vi "rvc Quadcopter Model.vi"(4 "tpp":dbl[](array[numeric]), 5 "d":dbl, 7 "b":dbl, 8 "omega4":dbl, 9 "omega3":dbl, 10 "omega2":dbl, 11 "omega1":dbl) -> (2 "tpp_2dot 2":dbl[](array[numeric]), 3 "xyz_2dot":dbl[](array[numeric]))   [LabVIEW 2013]
uses:
  <vilib>/imath/engines/lvmath2/RunTimeEngine/ErrorHandling/NIMS_Finalize Error.vi
  <vilib>/imath/engines/lvmath2/RunTimeEngine/Managers/WorkSpace/UID Generator.vi
  <vilib>/imath/engines/lvmath2/RunTimeEngine/Managers/SymbolTable/Clear UID.vi
  <vilib>/imath/engines/lvmath2/RunTimeEngine/NodeEndStatement/NIMS_NodeEndStatement_Output.vi
  <instcachedir>/0/NIMS_NodeEndStatement_Output_53EC0D466D134D7ABD903AC30B43404B.lvgen/NIMS_NodeEndStatement_Output_53EC0D466D134D7ABD903AC30B43404B_001.vi
  <vilib>/imath/engines/lvmath2/RunTimeEngine/RunTimeType/NIMS_RunTimeType_From StrictType (excl LVString).vi
  <instcachedir>/0/NIMS_RunTimeType_From StrictType (excl LVString)_4DEE718D6EB74582AA20236969C084FC.lvgen/NIMS_RunTimeType_From StrictType (excl LVString)_4DEE718D6EB74582AA20236969C084FC_000.vi
  <vilib>/imath/engines/lvmath2/RunTimeEngine/LocalVariableDefStatement/MC_LocalVariableDefStatement_Display.vi
  <vilib>/imath/engines/lvmath2/RunTimeEngine/Managers/SymbolTable/NIMS_WorkSpace.lvlib
panel:
  out "theta":dbl
  out "phi":dbl
  out "psi":dbl
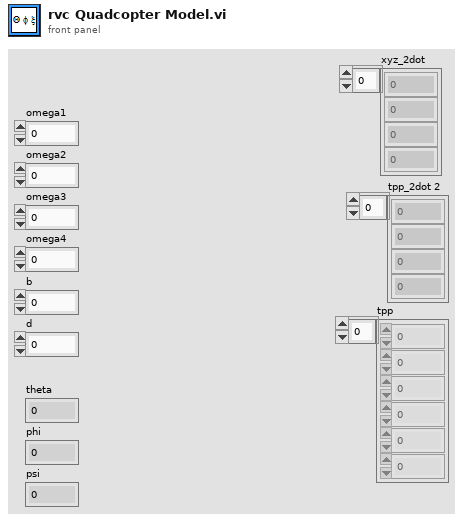
[diagram p1: front panel]
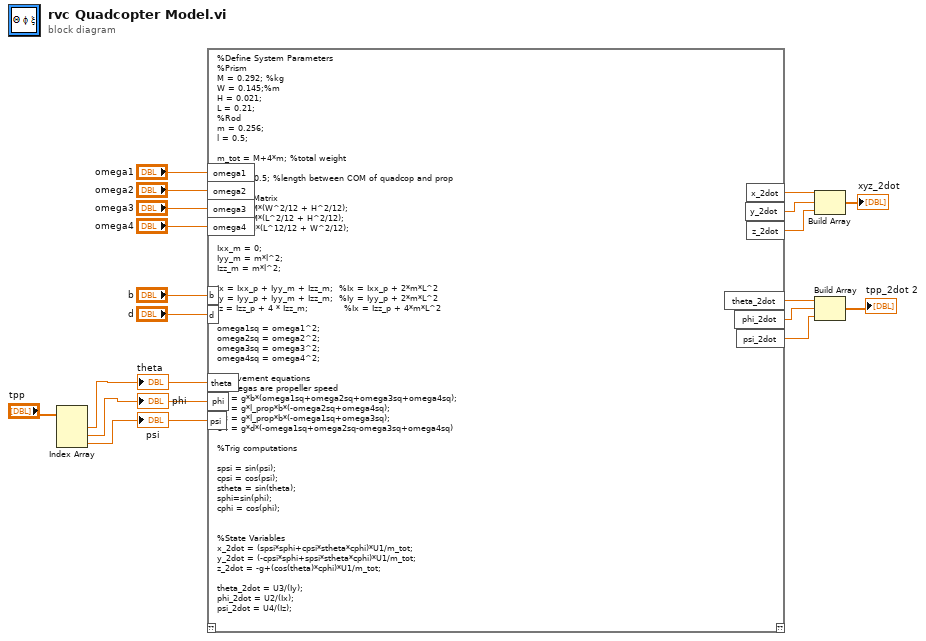
[diagram p0: block diagram]
diagram:
  n1 = Index Array(array="tpp") -> (element #1=w3:dbl, element #2=w2:dbl, element #3=w1:dbl)  [unwired: 3 in]
  "theta" <- w3
  "phi" <- w2
  "psi" <- w1
  n2 = mathscript code="%Define System Parameters\n%Prism\nM = 0.292; %kg\nW = 0.145;%m\nH = 0.021;\nL = 0.21;\n%Rod\nm = 0.256;\nl = 0.5;\n\nm_tot = M+4*m; %total weight\ng = 9.81;\nl_prop = 0.5; %length between COM of quadcop and prop\n\n%Inertia Matrix\nIxx_p = M*(W^2/12 + H^2/12);\nIyy_p = M*(L^2/12 + H^2/12);\nIzz_p = M*(L^12/12 + W^2/12);\n\nIxx_m = 0;\nIyy_m = m*l^2;\nIzz_m = m*l^2;\n\nIx = Ixx_p + Iyy_m + Izz_m;  %Ix = Ixx_p + 2*m*L^2\nIy = Iyy_p + Iyy_m + Izz_m;  %Iy = Iyy_p + 2*m*L^2\nIz = Izz_p + 4 * Izz_m;            %Ix = Izz_p + 4*m*L^2\n\nomega1sq = omega1^2;\nomega2sq = omega2^2;\nomega3sq = omega3^2;\nomega4sq = omega4^2;\n\n%Movement equations\n%omegas are propeller speed\nU1 = g*b*(omega1sq+omega2sq+omega3sq+omega4sq);\nU2 = g*l_prop*b*(-omega2sq+omega4sq);\nU3 = g*l_prop*b*(-omega1sq+omega3sq);\nU4 = g*d*(-omega1sq+omega2sq-omega3sq+omega4sq)\n\n%Trig computations\n\nspsi = sin(psi);\ncpsi = cos(psi);\nstheta = sin(theta);\nsphi=sin(phi);\ncphi = cos(phi);\n\n\n%State Variables\nx_2dot = (spsi*sphi+cpsi*stheta*cphi)*U1/m_tot;\ny_2dot = (-cpsi*sphi+spsi*stheta*cphi)*U1/m_tot;\nz_2dot = -g+(cos(theta)*cphi)*U1/m_tot;\n\ntheta_2dot = U3/(Iy);\nphi_2dot = U2/(Ix);\npsi_2dot = U4/(Iz);"("theta"=w3, "phi"=w2, "psi"=w1, "omega1"="omega1", "omega2"="omega2", "omega3"="omega3", "omega4"="omega4", "b"="b", "d"="d") -> ("x_2dot"=w12:dbl, "y_2dot"=w11:dbl, "z_2dot"=w10:dbl, "theta_2dot"=w9:dbl, "phi_2dot"=w8:dbl, "psi_2dot"=w7:dbl)  [unwired: 2 out]
  n3 = Build Array(w12, w11, w10) -> (→"xyz_2dot":dbl[])
  n4 = Build Array(w9, w8, w7) -> (→"tpp_2dot 2":dbl[])
